vi "Device.vi"(6 "Model":string, 7 "last calibration":string, 8 "error in (no error)":errorcluster caption="Fehler (Eingang, kein Fehler)", 9 "Hersteller":string, 10 "serial":string, 11 "Device Eingang":refnum<class "Device.lvclass"> caption="DNL_LabVIEW Object in") -> (0 "error out":errorcluster caption="Fehler (Ausgang)", 3 "Device Ausgang":refnum<class "Device.lvclass"> caption="DNL_LabVIEW Object out")   [LabVIEW 2013, in "DatenKlassen.lvlib" / "Device.lvclass"]
uses:
  Device.lvclass
  Device.lvclass/Device.ctl
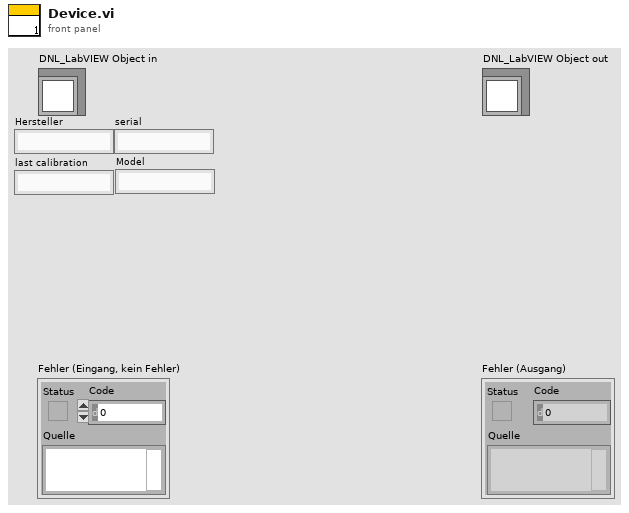
[diagram p1: front panel]
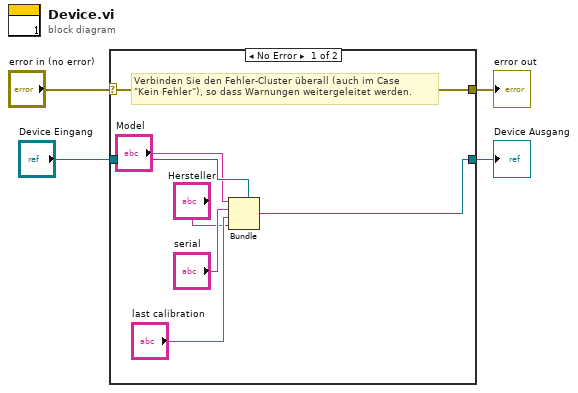
[diagram p0: block diagram]
diagram:
  n1 = case shown="No Error" "error in (no error)" {
    selector: "error in (no error)" -> [w11 w13]
    tunnel: [w11 w13] -> w3
    tunnel: [w7 w12] -> w1
    tunnel: "Device Eingang" -> [w8 w12]
    frame No Error {
      # "Verbinden Sie den Fehler-Cluster überall (auch im Case\n\"Kein Fehler\"), so dass Warnungen weitergeleitet werden."
      n2 = Bundle(cluster=w8, "Model", "serial", "last calibration", "Hersteller") -> (w7:refnum<class "Device.lvclass">)
    }
    frame Error {
    }
  }
  "error out" <- w3
  "Device Ausgang" <- w1
